vi "Receive.vi"(10 "Msg in":refnum<class "Msg.lvclass">, 11 "State in":refnum<class "State.lvclass">) -> (2 "Msg out":refnum<class "Msg.lvclass">)   [LabVIEW 2021, in "jettl.lvlib" / "jettl Queue Actor.lvlib" / "State.lvclass"]
uses:
  State.lvclass
  Actor/Msg/Msg.lvclass
panel:
  # "Connector Pane Note that Msg not object whose state we're altering, that is Queue Actor as seen in Handle and Teardown State methods."
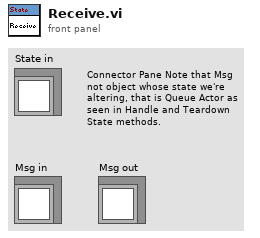
[diagram p1: front panel]
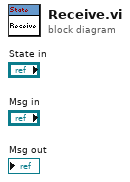
[diagram p0: block diagram]
diagram:
